vi "GyroActions.vi"(10 "Update?":bool, 11 "Zero":bool) -> (0 "Yaw":dbl, 3 "YRPHfH":T1)   [LabVIEW 2018]
uses:
  <vilib>/Rock Robotics/Network Tables/NT Read Boolean.vi
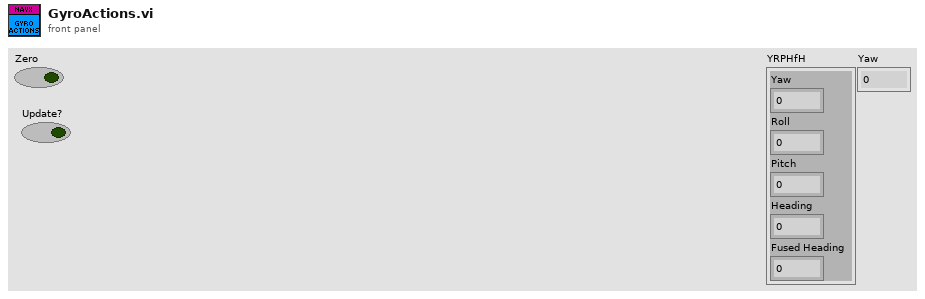
[diagram p1: front panel]
types:
  T1 = cluster{"Yaw":dbl, "Roll":dbl, "Pitch":dbl, "Heading":dbl, "Fused Heading":dbl}
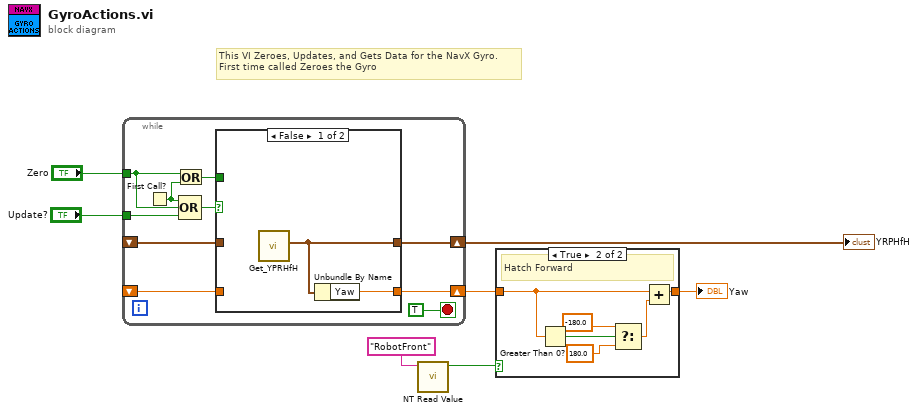
[diagram p0: block diagram]
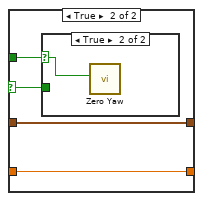
[diagram p3: hidden frame]
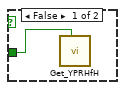
[diagram p4: hidden frame]
diagram:
  # "This VI Zeroes, Updates, and Gets Data for the NavX Gyro.\nFirst time called Zeroes the Gyro"
  n1 = while {
    tunnel: "Zero" -> [w14]
    tunnel: "Update?" -> [w13]
    shift-right: [w11] -> w5
    shift-left: _ -> [w9]
    shift-right: [w10] -> w3
    shift-left: _ -> [w8]
    stop <- TRUE stop-if-true
    n2 = First Call?() -> (First Call?: T/F=w15:bool)
    n3 = Or(x=w14, y=w15) -> (x .or. y?=w16:bool)
    n4 = Compound Arithmetic op=OR(w15, w14, w13) -> (w12:bool)
    n5 = case shown="False" w12 {
      selector: w12 -> [_ w22]
      tunnel: w16 -> [_ w23]
      tunnel: [w19 w21] -> w11
      tunnel: [w18 w20] -> w10
      tunnel: w9 -> [_ w21]
      tunnel: w8 -> [_ w20]
      frame False {
        n6 = call <vilib>:"Get_YPRHfH.vi"() -> ("YRPHfH"=w19:T1)  [unwired: 11 in]
        n7 = Unbundle By Name(w19) -> ("Yaw"=w18:dbl)
      }
      frame True {
        n8 = case shown="True" w23 {
          selector: w23 -> [_ w25]
          tunnel: w22 -> [w24 _]
          frame False {
            n9 = call <vilib>:"Get_YPRHfH.vi"("Update"=w24) -> ()  [unwired: 10 in, 1 out]
          }
          frame True {
            n10 = call <vilib>:"Zero Yaw.vi"("Zero"=w25) -> ()  [unwired: 11 in]
          }
        }
      }
    }
  }
  "YRPHfH" <- w5
  n11 = call-poly <vilib>:"NT Read Value.vi"("Name"="RobotFront") -> ("Boolean"=w2:bool)  [unwired: 9 in, 1 out]
  n12 = case shown="True" w2 {
    tunnel: [w26 w32] -> w4
    tunnel: w3 -> [w26 w31]
    frame False {
      # "Torros Forward"
    }
    frame True {
      # "Hatch Forward"
      n13 = Greater Than 0?(x=w31) -> (x > 0?=w30:bool)
      n14 = Select(t=-180.0, s=w30, f=180.0 ("y")) -> (s? t:f=w27:dbl)
      n15 = Add(x=w31, y=w27) -> (x+y=w32:dbl)
    }
  }
  "Yaw" <- w4
